vi "Pulsed BPSK Demodulator - channel 1.vi"() -> ()   [LabVIEW 2025]
uses:
  Program Files/NI/LVAddons/dltf/1/examples/Data Link Test Framework/Modems/Shared/BER/FPGA/PRBS/PRBS Degree Selection.ctl
  <vilib>/userDefined/High Color/nirio_resource_hc.ctl
  Support/Public/FPGA Refnum.ctl
  Program Files/NI/LVAddons/dltf/1/examples/Data Link Test Framework/Modems/Pulsed BPSK/Shared/Public/Demodulator Control.ctl
  Program Files/NI/LVAddons/dltf/1/examples/Data Link Test Framework/Modems/Shared/BER/Host/BER Host.lvclass
  <vilib>/addons/Modulation/Analog/controls/Complex Data Waveform.ctl
  cf92a2c4-daeb-48d3-813e-3e326d855d47.vi
  0254e0ab-5687-401b-9dc8-6f8770c9f38a.vi
  47a993e4-40c2-431a-96b5-958e41ced615.vi
  94b778db-892b-4d8c-b0b4-ded93cb94ed5.vi
  d2ae1a4e-c5da-4ddb-bfc0-d8bf5757701e.vi
  8e362640-a0be-4d2f-b44b-3cd6315c43a8.vi
  <vilib>/FPGAPlugInAG/Dynamic/niLvFpga_Download_Dynamic.vi
  <vilib>/FPGAPlugInAG/Dynamic/niLvFpga_Run_Dynamic.vi
  <vilib>/FPGAPlugInAG/Dynamic/niLvFpga_Close_Dynamic.vi
  <vilib>/rvi/interface/common/niFpgaWaitOnOcc.vi
  <vilib>/Utility/error.llb/Error Cluster From Error Code.vi
  <vilib>/rvi/errors/niLvFpgaAdjustHostInterfaceError.vi
  <vilib>/DLsc/v1/Host/Link Engine/Add Hardware - Single.vi
  <vilib>/DLsc/v1/Host/Protocols/Aurora 64b66b/Extension/Configure TX - Single.vi
  <vilib>/DLsc/v1/Host/Link Engine/Commit Links - Single.vi
  <vilib>/DLsc/v1/Host/Link Engine/Get Device Registers - IFW.vi
  <vilib>/DLsc/v1/Host/Link Engine/Enable Links - Single.vi
  <vilib>/DLsc/v1/Host/Link Engine/Abort Links - Single.vi
  <vilib>/DLsc/v1/Host/Link Engine/Disable Links - Single.vi
  <vilib>/DLsc/v1/Host/Link Engine/Close References - Single.vi
  <vilib>/rvi/interface/nirviMethod/nirviMethod.xnode
  <vilib>/rvi/interface/nirviCloseFPGA/nirviCloseFPGA.xnode
  <vilib>/rvi/interface/nirviReadWriteControl/nirviReadWriteControl.xnode
  <vilib>/rvi/interface/Simulation/niFpgaSimulationCallBeginRW.vi
  Support/Pulsed BPSK Host Support.lvlib
  <vilib>/FPGAPlugInAG/Dynamic/niLvFpga_ReadFifo_Dynamic.vi
  <vilib>/rvi/errors/niLvFpgaMergeErrorWithErrorCode.vi
  <vilib>/addons/Modulation/niDMT.lvlib
  Program Files/NI/LVAddons/dltf/1/examples/Data Link Test Framework/Modems/Shared/Modems Shared.lvlib
  Program Files/NI/LVAddons/dltf/1/examples/Data Link Test Framework/Modems/Pulsed BPSK/Shared/Pulsed BPSK Modem Shared.lvlib
  <vilib>/addons/Modulation/niAMT.lvlib
  Program Files/NI/LVAddons/dltf/1/examples/Data Link Test Framework/Modems/Shared/FIR/FIR.lvlib
  <vilib>/DLsc/v1/Host/Link Engine/DLsc Link Engine v1 Host.lvlib
  NiFpgaLv.dll
  <vilib>/DLsc/v1/Host/Protocols/Aurora 64b66b/Extension/Aurora 64b66b Extension.lvlib
  <vilib>/FPGAPlugInAG/Dynamic/niLvFpga_ConfigureFifo_Dynamic.vi
  <vilib>/FPGAPlugInAG/Dynamic/niLvFpga_StartFifo_Dynamic.vi
  Program Files/NI/LVAddons/dltf/1/examples/Data Link Test Framework/Modems/Shared/BER/FPGA/PRBS/PRBS.lvlib
panel:
  out "Constellation":T1(graph) caption="IQ Constellation"
  in  "Coprocessor Bitfile Path":path
  in  "Coprocessor Device Name":T2
  out "Bitfile Redownloaded":bool
  in  "Reset Demod":bool
  out "BER FPGA":dbl caption="Bit Error Rate" format="%.6f%%"
  in  "Signal Parameters":T4={"Symbol Rate (Hz)"=400000000.0, "Pulse Parameters"={"Payload Length"=800, "Preamble Symbol"=449838109, "PN Order"=4}} {"Pulse Parameters"."PN Order" items=["7", "9", "10", "11", "15", "17", "18", "20", "21", "22", "23", "25"]; "Pulse Parameters"."Preamble Symbol" format="%.0x"; "Symbol Rate (Hz)" format="%#_6p"}
  in  "Reset BER":bool
  out "Samples per Symbol":i32
  in  "stop":bool
  out "Status":string
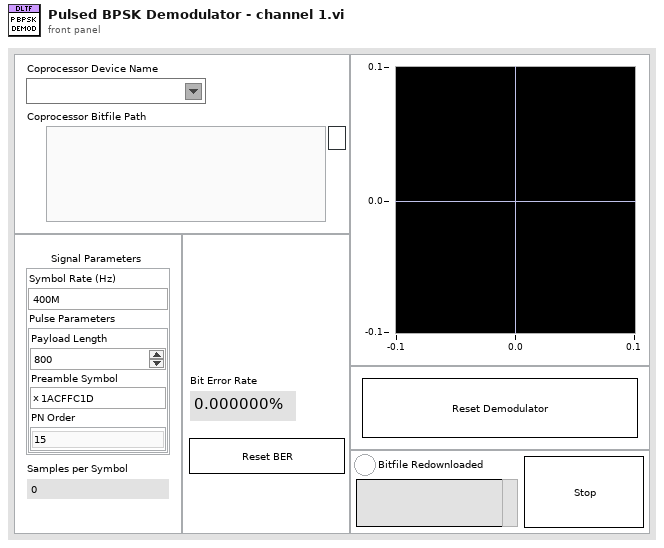
[diagram p1: front panel]
types:
  T1 = cluster{"constellation":dbl[], "oversampled data":dbl[]}[]
  T2 = typedef "nirio_resource_hc.ctl" = tag
  T3 = typedef "Modems Shared.lvlib/PRBS.lvlib/PRBS Degree Selection.ctl" = u16
  T4 = cluster{"Symbol Rate (Hz)":dbl, "Pulse Parameters":cluster{"Payload Length":u16, "Preamble Symbol":i32, "PN Order":T3}}
  T5 = typedef "Pulsed BPSK Modem Shared.lvlib/Demodulator Control.ctl" = i16
  T6 = typedef "Pulsed BPSK Host Support.lvlib/FPGA Refnum.ctl" = refnum<k20>
  T7 = typedef "DLsc Link Engine v1 Host.lvlib/DLsc Session.lvclass/Session Handle.ctl" = refnum<data-value>
  T8 = typedef "DLsc Link Engine v1 Host.lvlib/DLsc Session.lvclass/Device Address Information.ctl" = cluster{"device name":string, "bitfile path":path}
  T9 = cluster{"k1":fxp<+,17,-4>, "k2":fxp<+,17,-8>, "target level":fxp<+,18,2>, "level threshold":fxp<+,18,4>}
  T10 = cluster{"filter select":enum8{"None", "I Inline", "I Cross", "Q Cross", "Q Inline"}, "coef load":bool, "coef write":bool, "coef data":fxp<+/-,18,1>}
  T11 = typedef "niAMT.lvlib/Complex Data Waveform.ctl" = cluster{"t0":dbl, "dt":dbl, "Y":cdb[]}
  T12 = typedef "IFW Session v1 Host.lvlib/IFW Session.ctl" = cluster{"refnum":refnum<k20>, "subsystem map":refnum<class "niInstr Subsystem Map v1 Host.lvclass">, "register bus":refnum<class "niInstr FIFO Register Bus v1 Host.lvclass">, "IFW subsystems":T13}
  T13 = typedef "IFW Session v1 Host.lvlib/IFW Subsystems.ctl" = cluster{"IFW address space collection":T14}[]
  T14 = typedef "IFW Session v1 Host.lvlib/IFW Address Space Collection.ctl" = T15[]
  T15 = typedef "IFW Session v1 Host.lvlib/IFW Address Space.ctl" = cluster{"name":string, "IFW address space information":T16, "class path":path}
  T16 = typedef "IFW Session v1 Host.lvlib/IFW Address Space Information.ctl" = cluster{"UID":u16, "instance":u8}
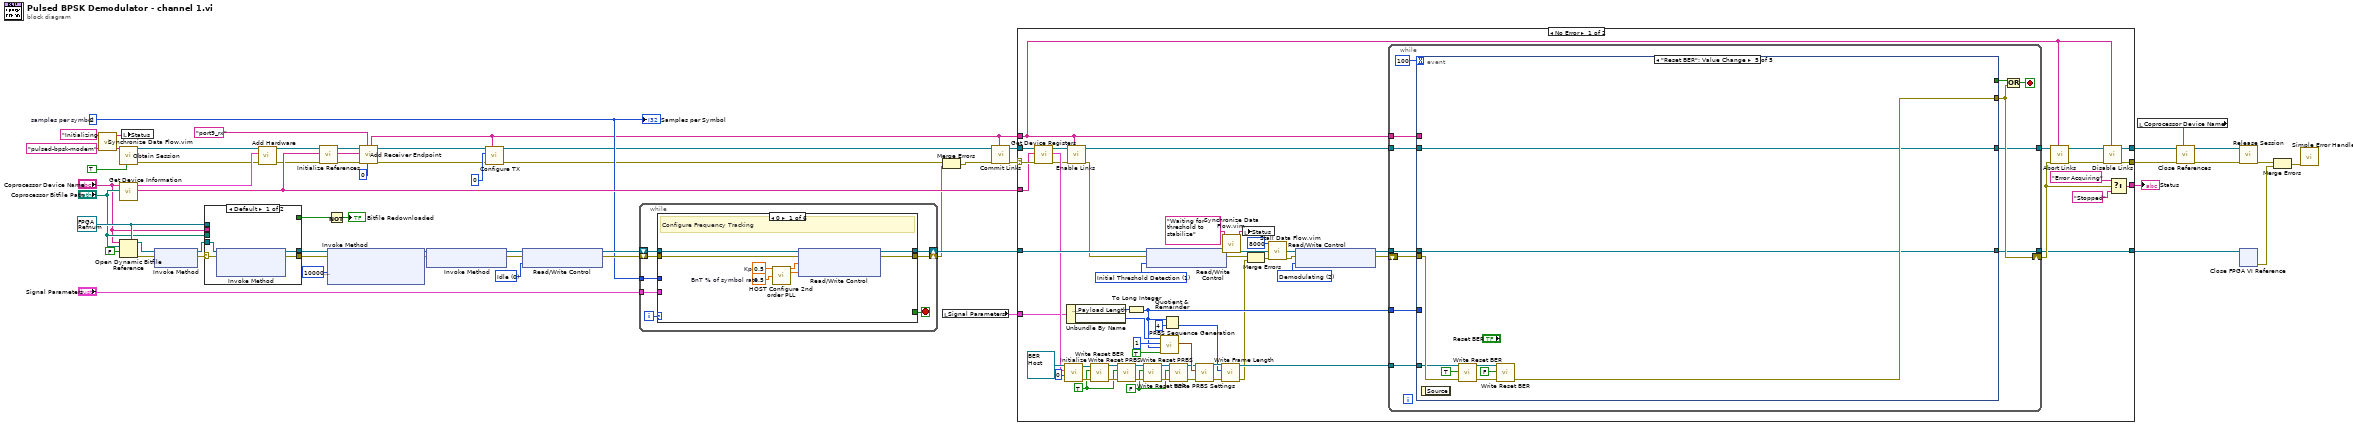
[diagram p0: block diagram]
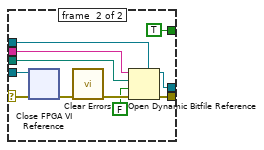
[diagram p2: hidden frame]
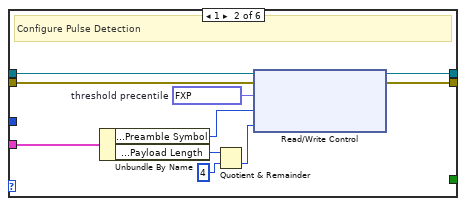
[diagram p3: hidden frame]
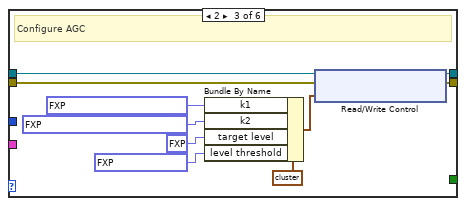
[diagram p4: hidden frame]
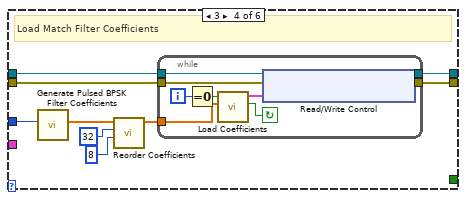
[diagram p5: hidden frame]
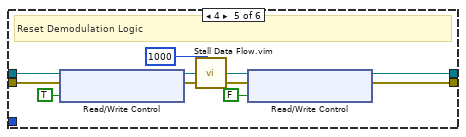
[diagram p6: hidden frame]
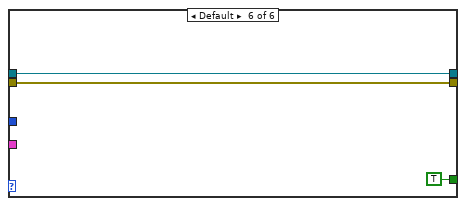
[diagram p7: hidden frame]
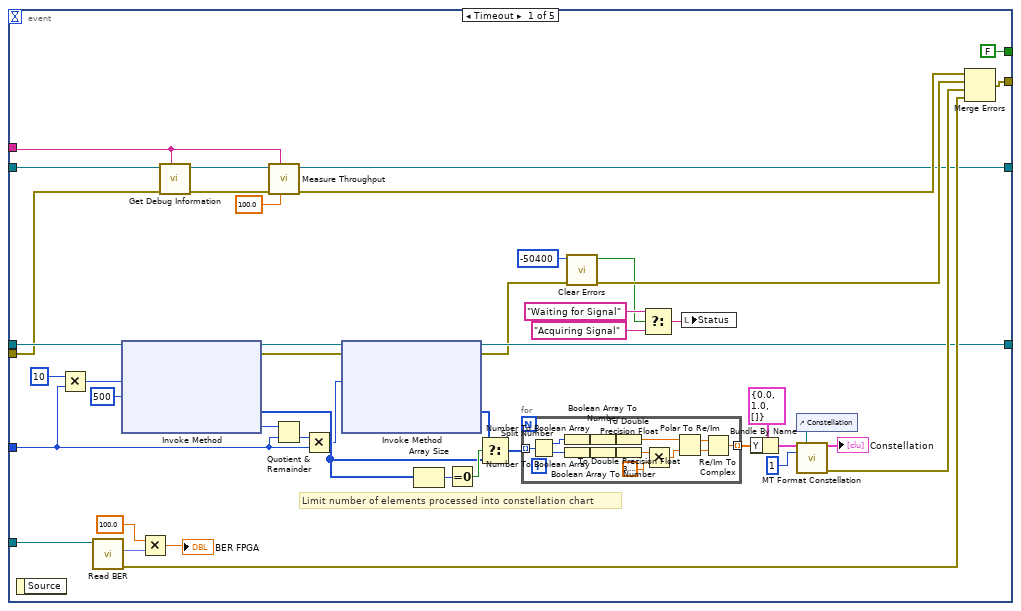
[diagram p8: hidden frame]
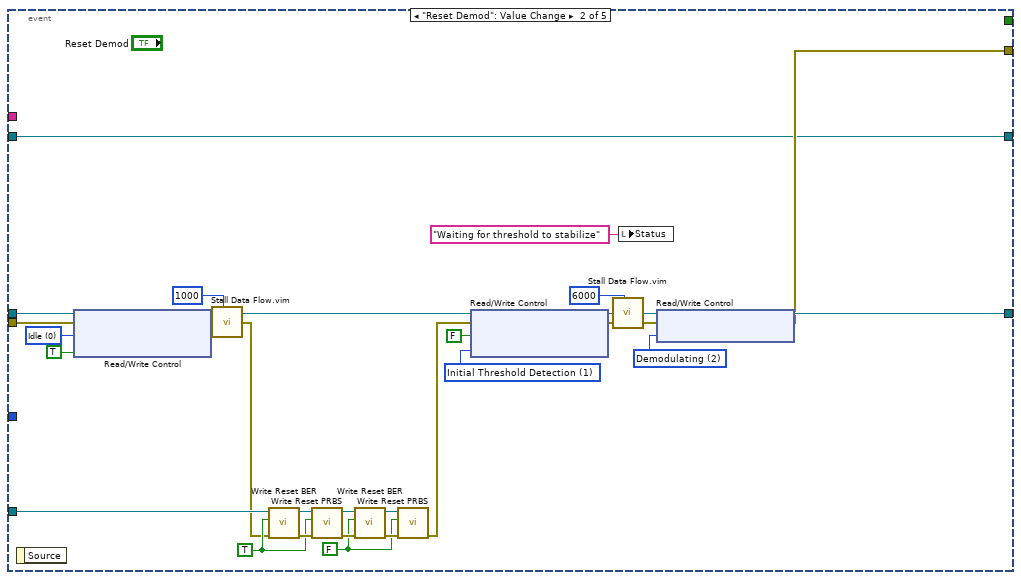
[diagram p9: hidden frame]
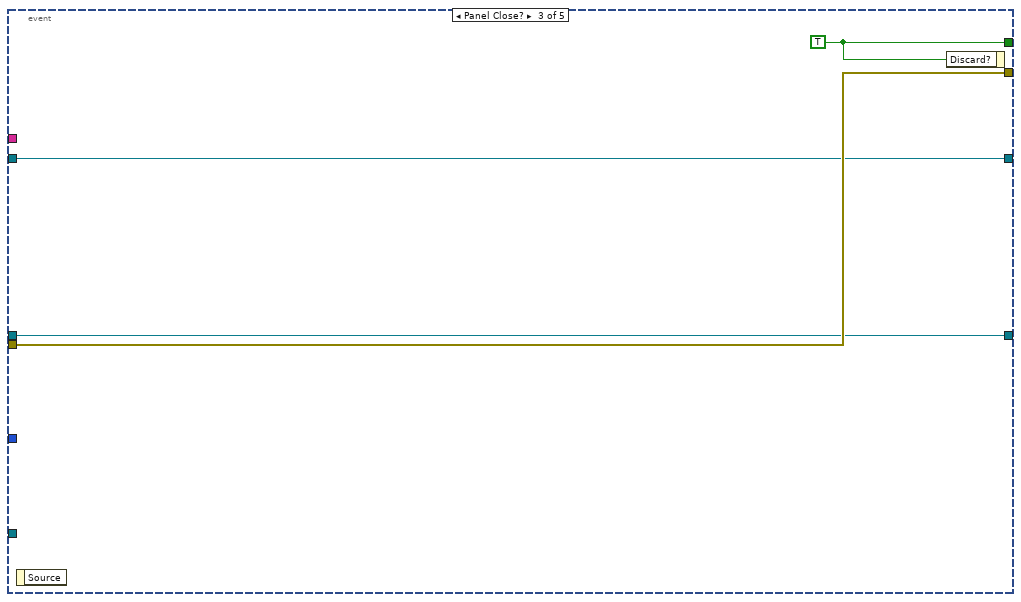
[diagram p10: hidden frame]
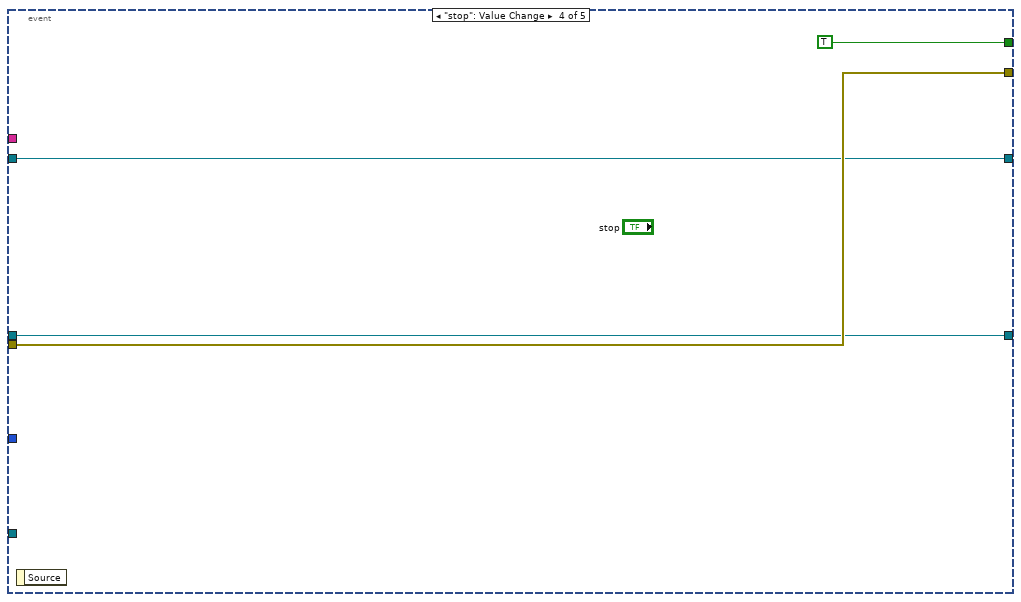
[diagram p11: hidden frame]
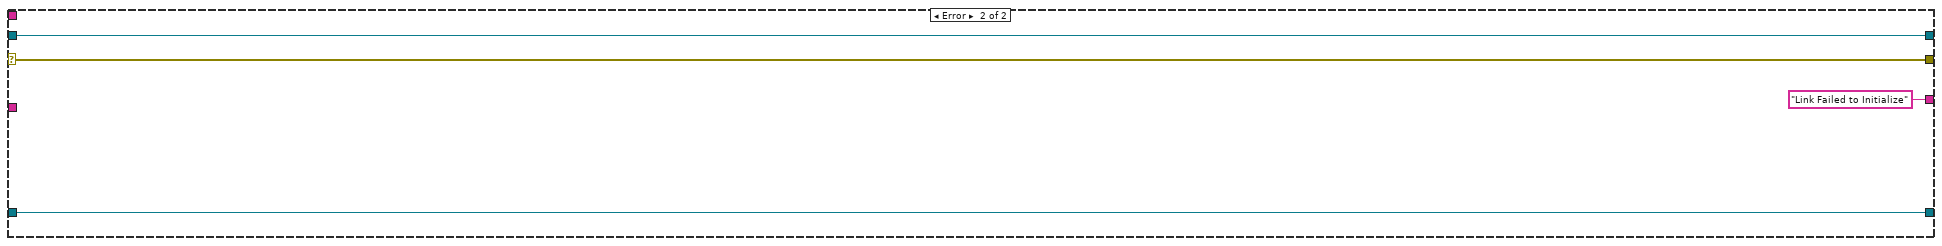
[diagram p12: hidden frame]
diagram:
  w47 = T5 0 items=["Idle", "Initial Threshold Detection", "Demodulating"] ("demodulator control")
  w21 = 2  # samples per symbol
  w31 = T6 refnum ("pulsed bpsk coprocessor refnum")
  n1 = call "Synchronize Data Flow.vim"("input 4"="pulsed-bpsk-modem", "input 1"="Initializing") -> ("output 4"=w27:string, "output 1"=w26:string)  [unwired: 2 in, 2 out]
  n2 = call <vilib>:"Obtain Session.vi"("use remote engine (f)"=TRUE ("Remote Engine"), "session name (\"\":default)"=w27) -> ("error out"=w13:errorcluster, "session out"=w14:T7)  [unwired: 6 in, 2 out]
  n3 = call <vilib>:"Get Device Information.vi"("bitfile path"="Coprocessor Bitfile Path", "device name"="Coprocessor Device Name") -> ("device name out"=w53:string, "device address information"=w52:T8)  [unwired: 7 in, 1 out]
  n4 = Open Dynamic Bitfile Reference(0:"Coprocessor Device Name", 1:"Coprocessor Bitfile Path", 2:FALSE ("Run When Loaded"), 4:w31) -> (5:w33:T6, 8:w32:errorcluster)  [unwired: 1 in]
  n5 = local write "Status"(w26) -> ()
  n6 = xnode "Invoke Method"("FPGA VI Reference In"=w33, "error in"=w32) -> ("FPGA VI Reference Out"=w36:T6, "error out"=w37:errorcluster)
  n7 = case shown="Default" w37 {
    selector: w37 -> [w61 w74]
    tunnel: [w63 w67] -> w34
    tunnel: [w62 w70] -> w35
    tunnel: w36 -> [w60 w72]
    tunnel: w31 -> [_ w68]
    tunnel: "Coprocessor Device Name" -> [_ w66]
    tunnel: "Coprocessor Bitfile Path" -> [_ w65]
    tunnel: [_ TRUE] -> w30
    frame #0 {
      n8 = xnode "Invoke Method"("FPGA VI Reference In"=w60, "error in"=w61) -> ("FPGA VI Reference Out"=w63:T6, "error out"=w62:errorcluster)  [unwired: 1 in]
    }
    frame #1 {
      n9 = xnode "Close FPGA VI Reference"("FPGA VI Reference In"=w72, "error in"=w74) -> ("error out"=w73:errorcluster)
      n10 = call <vilib>:"Clear Errors.vi"("error in (no error)"=w73) -> ("error out"=w71:errorcluster)  [unwired: 5 in, 1 out]
      n11 = Open Dynamic Bitfile Reference(0:w66, 1:w65, 2:FALSE ("Run When Loaded"), 3:w71, 4:w68) -> (5:w67:T6, 8:w70:errorcluster)
    }
  }
  n12 = call-poly <vilib>:"Add Hardware.vi"("error in"=w13, "device"=w52, "session in"=w14) -> ("error out"=w5:errorcluster, "session out"=w6:T7)  [unwired: 7 in]
  n13 = call <vilib>:"Initialize References.vi"("error in"=w5, "session in"=w6) -> ("error out"=w3:errorcluster, "session out"=w4:T7)  [unwired: 8 in]
  n14 = Not(x=w30) -> (.not. x?=→"Bitfile Redownloaded":bool)
  n15 = xnode "Invoke Method"("FPGA VI Reference In"=w34, "error in"=w35, "Requested Depth"=u32 100000000) -> ("FPGA VI Reference Out"=w41:T6, "error out"=w42:errorcluster)  [unwired: 1 out]
  n16 = call <vilib>:"Add Receiver Endpoint.vi"("receiver instance (0)"=u8 0, "link name"="port9_rx", "error in"=w3, "receiver device name"=w53, "session in"=w4) -> ("error out"=w1:errorcluster, "session out"=w2:T7, "link name out"=w10:string)  [unwired: 2 in, 2 out]
  n17 = xnode "Invoke Method"("FPGA VI Reference In"=w41, "error in"=w42) -> ("FPGA VI Reference Out"=w40:T6, "error out"=w39:errorcluster)
  n18 = call-poly <vilib>:"Configure TX.vi"("link name (\"\":default)"=w10, "error in"=w1, "frame size"=u16 0 ("tx frame size"), "session in"=w2) -> ("error out"=w7:errorcluster, "session out"=w8:T7)  [unwired: 6 in]
  n19 = xnode "Read/Write Control"("FPGA VI Reference In"=w40, "error in"=w39, "demodulator control.1"=w47) -> ("FPGA VI Reference Out"=w46:T6, "error out"=w48:errorcluster)
  n20 = while {
    shift-right: [w79] -> w44
    shift-left: w48 -> [w82]
    shift-right: [w80] -> w45
    shift-left: w46 -> [w81]
    tunnel: w21 -> [w76]
    tunnel: "Signal Parameters" -> [w75]
    i -> [w78]
    stop <- w77 stop-if-true
    n21 = case shown="0" w78 {
      tunnel: w82 -> [w86 w95 w110 w115 w137 w140]
      tunnel: w81 -> [w85 w94 w103 w114 w138 w141]
      tunnel: [w84 w93 w102 w113 w134 w141] -> w80
      tunnel: [w83 w92 w101 w112 w133 w140] -> w79
      tunnel: [_ _ _ _ _ TRUE] -> w77
      tunnel: w76 -> [_ _ _ w111 _ _]
      tunnel: w75 -> [_ w91 _ _ _ _]
      frame 0 {
        w90 = 0.5  # BnT % of symbol rate
        w89 = 0.5  # Kp
        # "Configure Frequency Tracking"
        n22 = call "HOST Configure 2nd order PLL.vi"("Kp"=w89, "BnT % of symbol rate"=w90) -> ("k1"=w88:dbl, "k2"=w87:dbl)  [unwired: 12 in]
        n23 = xnode "Read/Write Control"("FPGA VI Reference In"=w85, "error in"=w86, "frequency tracking k1.1"=w88, "frequency tracking k2.1"=w87) -> ("FPGA VI Reference Out"=w84:T6, "error out"=w83:errorcluster)
      }
      frame 1 {
        w100 = fxp<+/-,10,1> 0.701171875  # threshold precentile
        # "Configure Pulse Detection"
        n24 = Unbundle By Name(w91) -> ("Pulse Parameters.Preamble Symbol"=w97:i32, "Pulse Parameters.Payload Length"=w98:u16)
        n25 = Quotient & Remainder(x=w98, y=u16 4) -> (floor(x/y)=w96:u16)  [unwired: 1 out]
        n26 = xnode "Read/Write Control"("FPGA VI Reference In"=w94, "error in"=w95, "threshold precentile.1"=w100, "preamble.1"=w97, "frame length.1"=w96) -> ("FPGA VI Reference Out"=w93:T6, "error out"=w92:errorcluster)
      }
      frame 2 {
        # "Configure AGC"
        n27 = Bundle By Name(cluster=T9 {"k1"=0.0, "k2"=0.0, "target level"=0.0, "level threshold"=0.0} ("AGC configurations"), "k1"=fxp<+,17,-4> 0.03000020980834961, "k2"=fxp<+,17,-8> 0.0029999911785125732, "target level"=fxp<+,18,2> 0.5, "level threshold"=fxp<+,18,4> 0.0999755859375) -> (w104:T9)
        n28 = xnode "Read/Write Control"("FPGA VI Reference In"=w103, "error in"=w110, "AGC configurations.1"=w104) -> ("FPGA VI Reference Out"=w102:T6, "error out"=w101:errorcluster)
      }
      frame 3 {
        # "Load Match Filter Coefficients"
        n29 = call "Generate Pulsed BPSK Filter Coefficients.vi"("samples per symbol"=w111) -> ("pulse shaping filter coefficients"=w118:dbl[])  [unwired: 7 in, 3 out]
        n30 = call "Reorder Coefficients.vi"("spc"=8, "num taps"=32, "taps"=w118) -> ("reordered taps"=w119:dbl[])  [unwired: 8 in]
        n31 = while {
          tunnel: w114 -> [w127]
          tunnel: w115 -> [w126]
          tunnel: w119 -> [w128]
          tunnel: [w123] -> w113
          tunnel: [w122] -> w112
          i -> [w121]
          stop <- w124 continue-if-true
          n32 = Equal To 0?(x=w121) -> (x = 0?=w120:bool)
          n33 = call "Load Coefficients.vi"("coefficients"=w128, "load"=w120) -> ("loading"=w124:bool, "filter coefficients"=w125:T10)  [unwired: 8 in]
          n34 = xnode "Read/Write Control"("FPGA VI Reference In"=w127, "error in"=w126, "match filter coefficients.1"=w125) -> ("FPGA VI Reference Out"=w123:T6, "error out"=w122:errorcluster)
        }
      }
      frame 4 {
        # "Reset Demodulation Logic"
        n35 = xnode "Read/Write Control"("FPGA VI Reference In"=w138, "error in"=w137, "reset demodulator.1"=TRUE ("reset demodulator")) -> ("FPGA VI Reference Out"=w136:T6, "error out"=w135:errorcluster)
        n36 = call "Stall Data Flow.vim"("value in"=w136, "milliseconds to wait"=u32 1000) -> ("value out"=w130:T6)  [unwired: 1 out]
        n37 = xnode "Read/Write Control"("FPGA VI Reference In"=w130, "error in"=w135, "reset demodulator.1"=FALSE ("reset demodulator")) -> ("FPGA VI Reference Out"=w134:T6, "error out"=w133:errorcluster)
      }
      frame Default {
      }
    }
  }
  n38 = Merge Errors(w7, w44) -> (w9:errorcluster)
  n39 = local read "Signal Parameters"() -> (w25:T4)
  n40 = call-poly <vilib>:"Commit Links.vi"("link name (\"\":all)"=w10, "error in"=w9, "session in"=w8) -> ("error out"=w49:errorcluster, "session out"=w50:T7)  [unwired: 7 in]
  n41 = case shown="No Error" w49 {
    selector: w49 -> [w166 w319]
    tunnel: [w194 "Link Failed to Initialize" ("t")] -> w59
    tunnel: w50 -> [w167 w321]
    tunnel: w45 -> [w192 w320]
    tunnel: w10 -> [w152 _]
    tunnel: [w188 w321] -> w23
    tunnel: [w187 w320] -> w58
    tunnel: [w186 w319] -> w24
    tunnel: w53 -> [w162 _]
    tunnel: w25 -> [w161 _]
    frame No Error {
      w172 = FALSE ("reset")
      w171 = TRUE ("reset")
      w197 = T5 2 items=["Idle", "Initial Threshold Detection", "Demodulating"] ("demodulator control")
      w198 = T5 1 items=["Idle", "Initial Threshold Detection", "Demodulating"] ("demodulator control")
      n42 = call-poly <vilib>:"Get Device Registers.vi"("error in"=w166, "hardware name"=w162, "session in"=w167) -> ("error out"=w163:errorcluster, "ifw session"=w165:T12, "session out"=w164:T7)  [unwired: 6 in]
      n43 = call-dynamic "Initialize.vi"("instance(0)"=u8 0, "session"=w165, "ifw address space collection host in"=refnum<class "BER Host.lvclass"> refnum ("BER")) -> ("error out"=w177:errorcluster, "ifw address space collection host out"=w178:refnum<class "BER Host.lvclass">)  [unwired: 6 in, 1 out]
      n44 = Unbundle By Name(w161) -> ("Pulse Parameters.Payload Length"=w159:u16, "Pulse Parameters.PN Order"=w158:T3)
      n45 = call-poly <vilib>:"Enable Links.vi"("link name (\"\":all)"=w152, "error in"=w163, "session in"=w164) -> ("error out"=w144:errorcluster, "session out"=w151:T7)  [unwired: 7 in]
      n46 = call "Write Reset BER.vi"("error in"=w177, "reset"=w171, "BER"=w178) -> ("error out"=w181:errorcluster, "BER out"=w180:refnum<class "BER Host.lvclass">)  [unwired: 7 in]
      n47 = call "Write Reset PRBS.vi"("error in"=w181, "reset"=w171, "BER"=w180) -> ("error out"=w182:errorcluster, "BER out"=w183:refnum<class "BER Host.lvclass">)  [unwired: 7 in]
      n48 = To Long Integer(number=w159) -> (32bit integer=w155:i32)
      n49 = call "Write Reset BER.vi"("error in"=w182, "reset"=w172, "BER"=w183) -> ("error out"=w185:errorcluster, "BER out"=w184:refnum<class "BER Host.lvclass">)  [unwired: 7 in]
      n50 = xnode "Read/Write Control"("FPGA VI Reference In"=w192, "error in"=w144, "demodulator control.1"=w198) -> ("FPGA VI Reference Out"=w148:T6, "error out"=w149:errorcluster)
      n51 = call "PRBS Sequence Generation.vi"("backward"=TRUE, "total bits"=w155, "seed"=u32 1, "PRBS degree"=w158) -> ("PRBS setting"=w179:cluster{"degree":u8, "tap":u8, "seed":u32})  [unwired: 6 in, 1 out]
      n52 = Quotient & Remainder(x=w155, y=4) -> (floor(x/y)=w157:i32)  [unwired: 1 out]
      n53 = call "Write Reset PRBS.vi"("error in"=w185, "reset"=w172, "BER"=w184) -> ("error out"=w174:errorcluster, "BER out"=w173:refnum<class "BER Host.lvclass">)  [unwired: 7 in]
      n54 = call "Write PRBS Settings.vi"("error in"=w174, "PRBS Settings"=w179, "BER"=w173) -> ("error out"=w175:errorcluster, "BER out"=w176:refnum<class "BER Host.lvclass">)  [unwired: 7 in]
      n55 = call "Write Frame Length.vi"("error in"=w175, "frame length"=w157, "BER"=w176) -> ("error out"=w153:errorcluster, "BER out"=w168:refnum<class "BER Host.lvclass">)  [unwired: 7 in]
      n56 = call "Synchronize Data Flow.vim"("input 4"=w148, "input 1"="Waiting for threshold to stabilize" ("Status")) -> ("output 4"=w147:T6, "output 1"=w145:string)  [unwired: 2 in, 2 out]
      n57 = local write "Status"(w145) -> ()
      n58 = Merge Errors(w149, w153) -> (w154:errorcluster)
      n59 = call "Stall Data Flow.vim"("value in"=w147, "milliseconds to wait"=u32 8000) -> ("value out"=w150:T6)  [unwired: 1 out]
      n60 = xnode "Read/Write Control"("FPGA VI Reference In"=w150, "error in"=w154, "demodulator control.1"=w197) -> ("FPGA VI Reference Out"=w199:T6, "error out"=w200:errorcluster)
      n61 = while {
        shift-right: [w211] -> w189
        shift-left: w200 -> [w209]
        tunnel: w155 -> [w212]
        tunnel: w199 -> [w210]
        tunnel: w168 -> [w206]
        tunnel: w151 -> [w205]
        tunnel: [w204] -> w191
        tunnel: [w203] -> w187
        tunnel: w152 -> [w202]
        stop <- w201 stop-if-true
        n62 = event shown="[4] \"Reset BER\": Value Change" {
          selector: _ -> [_ _ _ _ _]
          dyn-events: _ -> [_ _ _ _ _]
          timeout: 100 -> [_ _ _ _ _]
          tunnel: w212 -> [w243 _ _ _ _]
          tunnel: [w257 w284 w304 w307 w311] -> w211
          tunnel: w210 -> [w240 w300 w301 w305 w309]
          tunnel: w209 -> [w219 w279 w304 w307 w317]
          tunnel: [FALSE ("stop") _ w303 TRUE ("stop") _] -> w208
          tunnel: w206 -> [w247 w288 _ _ w316]
          tunnel: w205 -> [w220 w280 w302 w306 w310]
          tunnel: [w217 w280 w302 w306 w310] -> w204
          tunnel: [w238 w286 w301 w305 w309] -> w203
          tunnel: w202 -> [w221 _ _ _ _]
          event Timeout {
            # "Limit number of elements processed into constellation chart"
            n63 = event-data() -> ()  [unwired: 1 in, 1 out]
            n64 = Multiply(x=u32 10 ("Data Fetch Multiplier"), y=w243) -> (x*y=w216:u32)
            n65 = call "Read BER.vi"("BER"=w247) -> ("error out"=w239:errorcluster, "BER"=w245:fxp<+,32,0>)  [unwired: 8 in, 1 out]
            n66 = xnode "Invoke Method"("FPGA VI Reference In"=w240, "Number of Elements"=w216, "Timeout (ms)"=500) -> ("FPGA VI Reference Out"=w242:T6, "error out"=w235:errorcluster, "Data"=w228:u32[], "Elements Remaining"=w227:u32)  [unwired: 1 in]
            n67 = Multiply(x=100.0, y=w245) -> (x*y=→"BER FPGA":dbl)
            n68 = call <vilib>:"Get Debug Information.vi"("link name"=w221, "error in"=w219, "session in"=w220) -> ("error out"=w224:errorcluster, "session out"=w223:T7)  [unwired: 5 in, 2 out]
            n69 = call <vilib>:"Measure Throughput.vi"("measurement interval (500ms)"=100.0 ("thruput meas time (ms)"), "link name"=w221, "error in"=w224, "session in"=w223) -> ("error out"=w218:errorcluster, "session out"=w217:T7)  [unwired: 4 in, 2 out]
            n70 = Quotient & Remainder(x=w227, y=w243) -> (floor(x/y)=w241:u32)  [unwired: 1 out]
            n71 = Multiply(x=w241, y=w243) -> (x*y=w214:u32)
            n72 = xnode "Invoke Method"("FPGA VI Reference In"=w242, "error in"=w235, "Number of Elements"=w214) -> ("FPGA VI Reference Out"=w238:T6, "error out"=w237:errorcluster, "Data"=w226:u32[])  [unwired: 1 in, 1 out]
            n73 = Array Size(array=w228) -> (size(s)=w234:i32)
            n74 = Equal To 0?(x=w234) -> (x = 0?=w233:bool)
            n75 = Select(t=w226, s=w233, f=w228) -> (s? t:f=w215:u32[])
            n76 = for {
              tunnel: w215 -> [w271] mode=indexing
              tunnel: [w264] -> w256 mode=indexing
              n77 = Split Number(x=w271) -> (hi(x)=w270:u16, lo(x)=w269:u16)
              n78 = Number To Boolean Array(number=w270) -> (Boolean array=w268:bool[])
              n79 = Number To Boolean Array(number=w269) -> (Boolean array=w267:bool[])
              n80 = Boolean Array To Number(Boolean array=w268) -> (number=w266:fxp<+/-,16,2>)
              n81 = Boolean Array To Number(Boolean array=w267) -> (number=w265:fxp<+/-,16,1>)
              n82 = To Double Precision Float(number=w266) -> (double precision float=w260:dbl)
              n83 = To Double Precision Float(number=w265) -> (double precision float=w261:dbl)
              n84 = Multiply(x=w261, y=3.141592653589793) -> (x*y=w263:dbl)
              n85 = Polar To Re/Im(2:w263, 3:w260) -> (0:w259:dbl, 1:w258:dbl)
              n86 = Re/Im To Complex(1:w259, 2:w258) -> (0:w264:cdb)
            }
            n87 = call <vilib>:"Clear Errors.vi"("error in (no error)"=w237, "specific error code to clear (0: all)"=-50400) -> ("error out"=w232:errorcluster, "specific error cleared?"=w231:bool)  [unwired: 4 in]
            n88 = Select(t="Waiting for Signal", s=w231, f="Acquiring Signal") -> (s? t:f=w248:string)
            n89 = local write "Status"(w248) -> ()
            n90 = Bundle By Name(cluster=T11 {"t0"=0.0, "dt"=1.0, "Y"=[]} ("waveform"), "Y"=w256) -> (w251:T11)
            n91 = control-ref of="Constellation"() -> (w229:refnum<vi>)
            n92 = call <vilib>:"MT Format Constellation.vi"("waveform"=w251, "constellation reference"=w229, "samples per symbol"=1) -> ("constellation graph"=→"Constellation":T1, "error out"=w254:errorcluster)  [unwired: 2 in, 9 out]
            n93 = Merge Errors(w218, w232, w254, w239) -> (w257:errorcluster)
          }
          event "Reset Demod": Value Change {
            w277 = T5 1 items=["Idle", "Initial Threshold Detection", "Demodulating"] ("demodulator control")
            w285 = T5 2 items=["Idle", "Initial Threshold Detection", "Demodulating"] ("demodulator control")
            w290 = FALSE ("reset")
            w289 = TRUE ("reset")
            w299 = T5 0 items=["Idle", "Initial Threshold Detection", "Demodulating"] ("demodulator control")
            n94 = event-data() -> ()  [unwired: 1 in, 1 out]
            n95 = xnode "Read/Write Control"("FPGA VI Reference In"=w300, "error in"=w279, "demodulator control.1"=w299, "reset demodulator.1"=TRUE ("reset demodulator")) -> ("FPGA VI Reference Out"=w283:T6, "error out"=w282:errorcluster)
            n96 = call "Stall Data Flow.vim"("value in"=w282, "milliseconds to wait"=u32 1000) -> ("value out"=w281:errorcluster)  [unwired: 1 out]
            n97 = call "Write Reset BER.vi"("error in"=w281, "reset"=w289, "BER"=w288) -> ("error out"=w292:errorcluster, "BER out"=w291:refnum<class "BER Host.lvclass">)  [unwired: 7 in]
            n98 = call "Write Reset PRBS.vi"("error in"=w292, "reset"=w289, "BER"=w291) -> ("error out"=w293:errorcluster, "BER out"=w294:refnum<class "BER Host.lvclass">)  [unwired: 7 in]
            n99 = call "Write Reset BER.vi"("error in"=w293, "reset"=w290, "BER"=w294) -> ("error out"=w296:errorcluster, "BER out"=w295:refnum<class "BER Host.lvclass">)  [unwired: 7 in]
            n100 = call "Write Reset PRBS.vi"("error in"=w296, "reset"=w290, "BER"=w295) -> ("error out"=w287:errorcluster)  [unwired: 7 in, 1 out]
            n101 = xnode "Read/Write Control"("FPGA VI Reference In"=w283, "error in"=w287, "reset demodulator.1"=FALSE ("reset modulator"), "demodulator control.1"=w277) -> ("FPGA VI Reference Out"=w276:T6, "error out"=w275:errorcluster)
            n102 = call "Stall Data Flow.vim"("value in"=w276, "milliseconds to wait"=u32 6000) -> ("value out"=w274:T6)  [unwired: 1 out]
            n103 = local write "Status"("Waiting for threshold to stabilize" ("Status")) -> ()
            n104 = xnode "Read/Write Control"("FPGA VI Reference In"=w274, "error in"=w275, "demodulator control.1"=w285) -> ("FPGA VI Reference Out"=w286:T6, "error out"=w284:errorcluster)
          }
          event Panel Close? {
            w303 = TRUE ("stop")
            n105 = event-data() -> ()  [unwired: 1 in, 1 out]
            n106 = event-data("Discard?"=w303) -> ()  [unwired: 1 in, 1 out]
          }
          event "stop": Value Change {
            n107 = event-data() -> ()  [unwired: 1 in, 1 out]
          }
          event "Reset BER": Value Change {
            n108 = event-data() -> ()  [unwired: 1 in, 1 out]
            n109 = call "Write Reset BER.vi"("error in"=w317, "reset"=TRUE, "BER"=w316) -> ("error out"=w314:errorcluster, "BER out"=w313:refnum<class "BER Host.lvclass">)  [unwired: 7 in]
            n110 = call "Write Reset BER.vi"("error in"=w314, "reset"=FALSE, "BER"=w313) -> ("error out"=w311:errorcluster)  [unwired: 7 in, 1 out]
          }
        }
        n111 = Or(x=w208, y=w211) -> (x .or. y?=w201:bool)
      }
      n112 = call-poly <vilib>:"Abort Links.vi"("link name (\"\":all)"=w152, "error in"=w189, "session in"=w191) -> ("error out"=w143:errorcluster, "session out"=w190:T7)  [unwired: 7 in]
      n113 = call-poly <vilib>:"Disable Links.vi"("link name (\"\":all)"=w152, "error in"=w143, "session in"=w190) -> ("error out"=w186:errorcluster, "session out"=w188:T7)  [unwired: 7 in]
      n114 = Select(t="Error Acquiring", s=w189, f="Stopped") -> (s? t:f=w194:string)
    }
    frame Error {
    }
  }
  "Status" <- w59
  n115 = local read "Coprocessor Device Name"() -> (w22:T2)
  n116 = call-poly <vilib>:"Close References.vi"("device name"=w22, "error in"=w24, "session in"=w23) -> ("error out"=w16:errorcluster, "session out"=w17:T7)  [unwired: 7 in]
  n117 = call <vilib>:"Release Session.vi"("error in"=w16, "session in"=w17) -> ("error out"=w57:errorcluster)  [unwired: 8 in, 1 out]
  n118 = xnode "Close FPGA VI Reference"("FPGA VI Reference In"=w58) -> ("error out"=w20:errorcluster)  [unwired: 1 in]
  n119 = Merge Errors(w57, w20) -> (w56:errorcluster)
  n120 = call <vilib>:"Simple Error Handler.vi"("error in (no error)"=w56) -> ()  [unwired: 4 in, 5 out]
  "Samples per Symbol" <- w21
